vi "close.vi"(8 "error in (no error)":errorcluster, 11 "Camera in":refnum<class "Camera.lvclass">) -> (0 "error out":errorcluster)   [LabVIEW 2019, in "Camera.lvclass"]
doc: "Closes the activated camera and releases the blocked ressources. This function must be called\nbefore the application is terminated. Otherwise, the resources remain occupied."
uses:
  Camera.lvclass
  pco.convert/Convert.lvlib
  pco.sdk/LensControl/LensControl.lvlib
  pco.recorder/Recorder.lvlib
  pco.sdk/CameraAccess/CameraAccess.lvlib
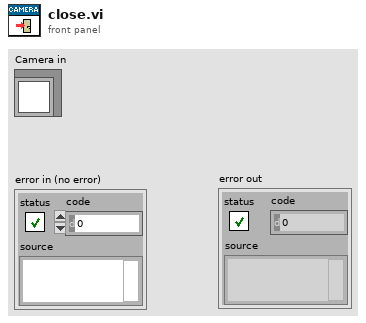
[diagram p1: front panel]
types:
  T1 = enum16{"Undefined", "Mono8", "Mono16", "BGRA8", "RGBA8", "BGRA16", "RGBA16", "CompressedMono8"}
  T2 = map{enum16{"Undefined", "Mono8", "Mono16", "BGRA8", "RGBA8", "BGRA16", "RGBA16", "CompressedMono8"}, u64}
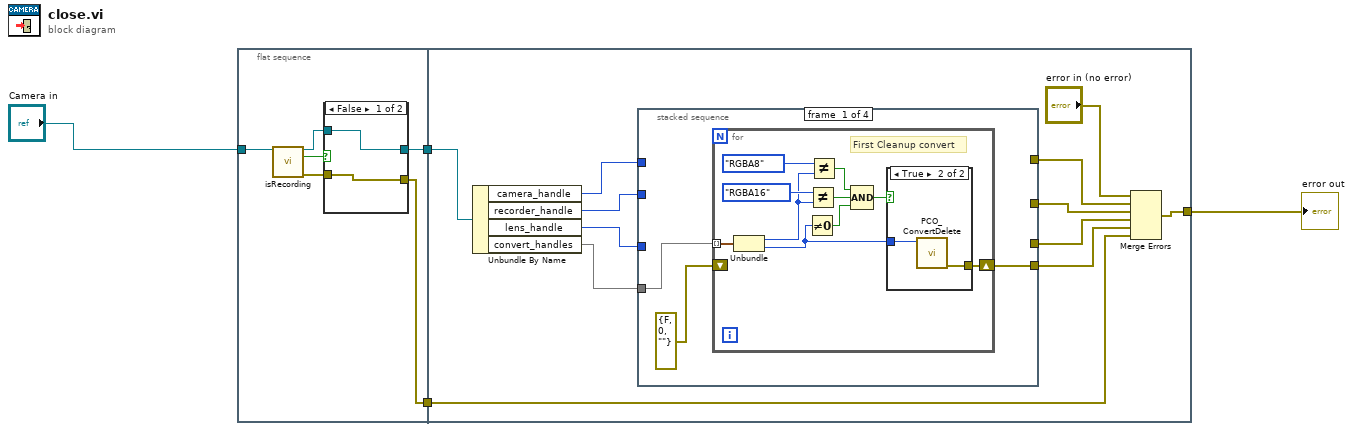
[diagram p0: block diagram]
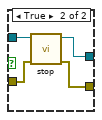
[diagram p2: hidden frame]
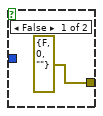
[diagram p3: hidden frame]
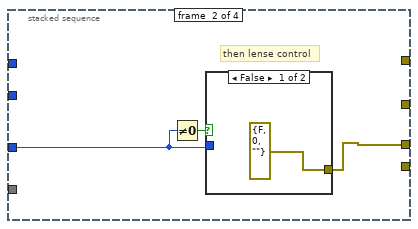
[diagram p4: hidden frame]
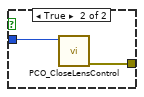
[diagram p5: hidden frame]
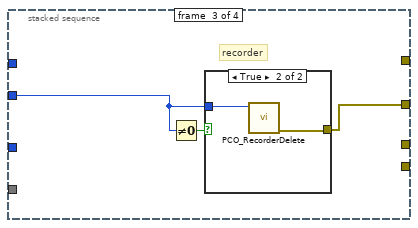
[diagram p6: hidden frame]
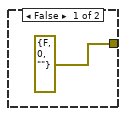
[diagram p7: hidden frame]
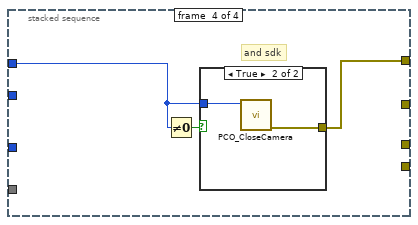
[diagram p8: hidden frame]
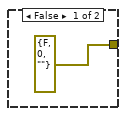
[diagram p9: hidden frame]
diagram:
  n1 = flat-sequence {
    tunnel: "Camera in" -> [w10]
    tunnel: [w6] -> w2
    tunnel: [w5] -> w1
    tunnel: [w21] -> w4
    tunnel: w2 -> [w20]
    tunnel: w1 -> [w17]
    frame #0 {
      n2 = call-dynamic "isRecording.vi"("Camera in"=w10) -> ("Camera out"=w8:refnum<class "Camera.lvclass">, "recording"=w9:bool, "error out"=w7:errorcluster)  [unwired: 12 in]
      n3 = case shown="False" w9 {
        tunnel: w8 -> [w12 w16]
        tunnel: w7 -> [w11 w15]
        tunnel: [w12 w14] -> w6
        tunnel: [w11 w13] -> w5
        frame False {
        }
        frame True {
          n4 = call-dynamic "stop.vi"("error in (no error)"=w15, "Camera in"=w16) -> ("error out"=w13:errorcluster, "Camera out"=w14:refnum<class "Camera.lvclass">)  [unwired: 8 in]
        }
      }
    }
    frame #1 {
      n5 = Unbundle By Name(w20) -> ("camera_handle"=w26:u64, "recorder_handle"=w27:u64, "lens_handle"=w28:u64, "convert_handles"=w19:T2)
      n6 = stacked-sequence {
        tunnel: w19 -> [w29 _ _ _]
        tunnel: w28 -> [_ w46 _ _]
        tunnel: w27 -> [_ _ w52 _]
        tunnel: w26 -> [_ _ _ w57]
        tunnel: [w31 _ _ _] -> w22
        tunnel: [_ w45 _ _] -> w23
        tunnel: [_ _ w51 _] -> w24
        tunnel: [_ _ _ w58] -> w25
        frame #0 {
          n7 = for {
            shift-right: [w41] -> w31
            shift-left: errorcluster {"status"=FALSE, "code"=0, "source"=""} ("error out") -> [_]
            tunnel: w29 -> [w40] mode=indexing
            # "First Cleanup convert"
            n8 = Unbundle(w40) -> (w36:T1, w37:u64)
            n9 = Not Equal To 0?(x=w37) -> (x != 0?=w33:bool)
            n10 = Not Equal?(x=T1."RGBA16", y=w36) -> (x != y?=w34:bool)
            n11 = Not Equal?(x=T1."RGBA8", y=w36) -> (x != y?=w35:bool)
            n12 = Compound Arithmetic op=AND(w35, w34, w33) -> (w32:bool)
            n13 = case shown="True" w32 {
              tunnel: w37 -> [_ w43]
              tunnel: [errorcluster {"status"=FALSE, "code"=0, "source"=""} ("error out") w44] -> w41
              frame False {
              }
              frame True {
                n14 = call "PCO_ConvertDelete.vi"("ph"=w43) -> ("error out"=w44:errorcluster)  [unwired: 9 in, 1 out]
              }
            }
          }
        }
        frame #1 {
          # "then lense control"
          n15 = Not Equal To 0?(x=w46) -> (x != 0?=w47:bool)
          n16 = case shown="False" w47 {
            tunnel: w46 -> [_ w50]
            tunnel: [errorcluster {"status"=FALSE, "code"=0, "source"=""} ("error out") w49] -> w45
            frame False {
            }
            frame True {
              n17 = call "PCO_CloseLensControl.vi"("hLens"=w50) -> ("error out"=w49:errorcluster)  [unwired: 9 in, 1 out]
            }
          }
        }
        frame #2 {
          # "recorder"
          n18 = Not Equal To 0?(x=w52) -> (x != 0?=w53:bool)
          n19 = case shown="True" w53 {
            tunnel: [errorcluster {"status"=FALSE, "code"=0, "source"=""} ("error out") w56] -> w51
            tunnel: w52 -> [_ w55]
            frame False {
            }
            frame True {
              n20 = call "PCO_RecorderDelete.vi"("phRec"=w55) -> ("error out"=w56:errorcluster)  [unwired: 9 in, 1 out]
            }
          }
        }
        frame #3 {
          # "and sdk"
          n21 = Not Equal To 0?(x=w57) -> (x != 0?=w59:bool)
          n22 = case shown="True" w59 {
            tunnel: [errorcluster {"status"=FALSE, "code"=0, "source"=""} ("error out") w62] -> w58
            tunnel: w57 -> [_ w61]
            frame False {
            }
            frame True {
              n23 = call "PCO_CloseCamera.vi"("ph"=w61) -> ("error out"=w62:errorcluster)  [unwired: 9 in, 1 out]
            }
          }
        }
      }
      n24 = Merge Errors("error in (no error)", w25, w24, w23, w22, w17) -> (w21:errorcluster)
    }
  }
  "error out" <- w4
